vi "Unary ni_measurements_discovery_v1_RegistryService_RegisterService.vi"(8 "error in":errorcluster, 10 "Request Data":T2, 11 "gRPC ID":T5) -> (0 "error out":errorcluster, 2 "Response Data":T1, 3 "gRPC ID out":T5)   [LabVIEW 2020, in "Discovery_client.lvlib"]
uses:
  Discovery_client.lvlib
  <vilib>/gRPC/LabVIEW gRPC Library/Server API/typeDefs/grpcId.ctl
  RPC Messages/ni_measurements_discovery_v1_RegisterServiceRequest.ctl
  RPC Messages/ni_measurements_discovery_v1_ServiceDescriptor.ctl
  RPC Messages/ni_measurements_discovery_v1_ServiceLocation.ctl
  RPC Messages/ni_measurements_discovery_v1_RegisterServiceResponse.ctl
  3477ff3c-ac1a-41b2-98e0-1f89dff8fa77.vi
  <vilib>/gRPC/LabVIEW gRPC Library/Server API/Server/Get Server DLL Path.vi
  <vilib>/gRPC/LabVIEW gRPC Library/Server API/TranslateGrpcError.vi
  <vilib>/gRPC/LabVIEW gRPC Library/gprc-lvsupport-release.lvlib
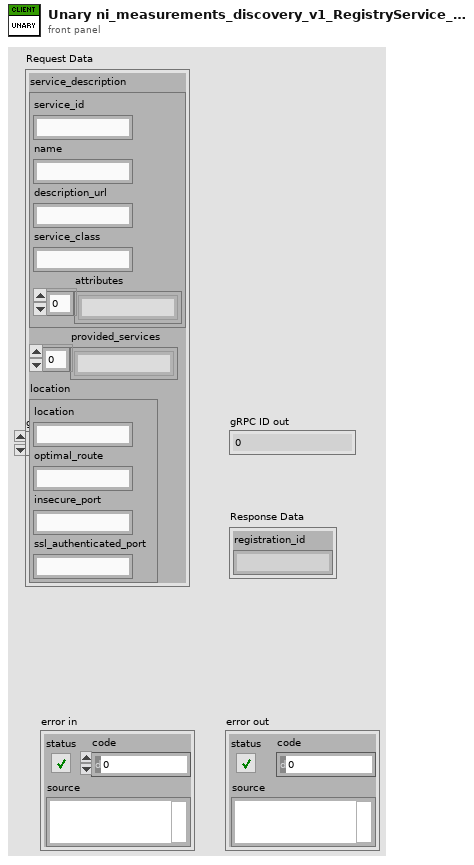
[diagram p1: front panel]
types:
  T1 = typedef "Discovery_client.lvlib/ni_measurements_discovery_v1_RegisterServiceResponse.ctl" = cluster{"registration_id":string}
  T2 = typedef "Discovery_client.lvlib/ni_measurements_discovery_v1_RegisterServiceRequest.ctl" = cluster{"service_description":T3, "provided_services":string[], "location":T4}
  T3 = typedef "Discovery_client.lvlib/ni_measurements_discovery_v1_ServiceDescriptor.ctl" = cluster{"service_id":string, "name":string, "description_url":string, "service_class":string, "attributes":string[]}
  T4 = typedef "Discovery_client.lvlib/ni_measurements_discovery_v1_ServiceLocation.ctl" = cluster{"location":string, "optimal_route":string, "insecure_port":string, "ssl_authenticated_port":string}
  T5 = typedef "gprc-lvsupport-release.lvlib/grpcId.ctl" = u64
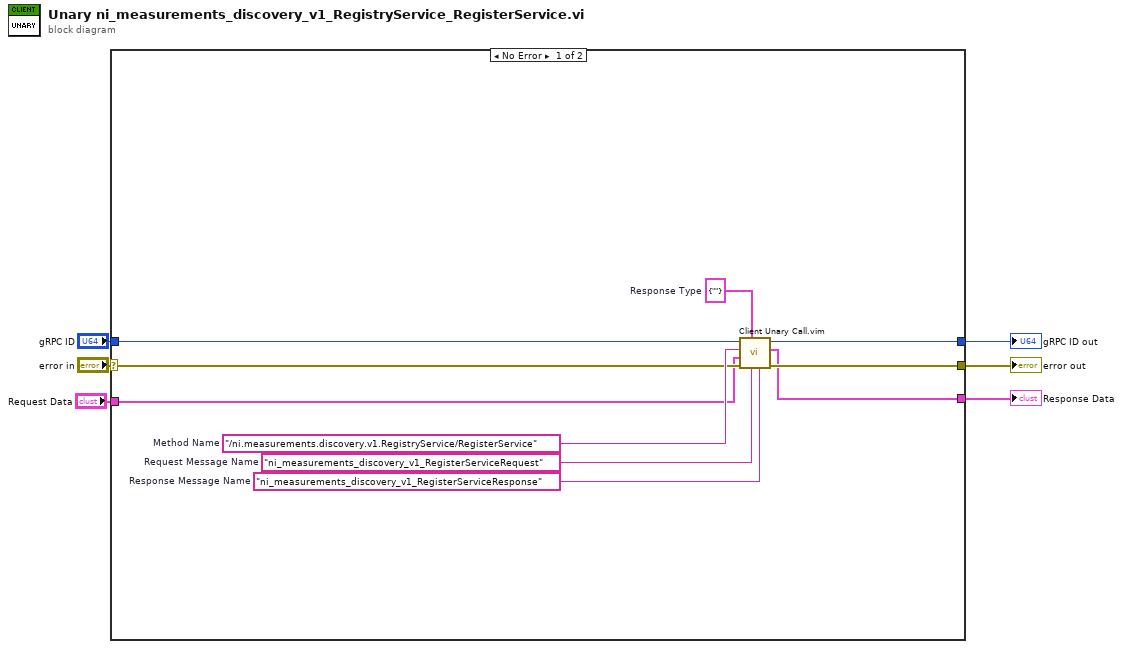
[diagram p0: block diagram]
diagram:
  n1 = case shown="No Error" "error in" {
    selector: "error in" -> [w12 w17]
    tunnel: [w11 w17] -> w5
    tunnel: "gRPC ID" -> [w10 w18]
    tunnel: [w9 w18] -> w3
    tunnel: "Request Data" -> [w8 _]
    tunnel: [w7 _] -> w1
    frame No Error {
      w13 = "ni_measurements_discovery_v1_RegisterServiceResponse"  # Response Message Name
      w14 = "ni_measurements_discovery_v1_RegisterServiceRequest"  # Request Message Name
      w15 = T1 {"registration_id"=""}  # Response Type
      w16 = "/ni.measurements.discovery.v1.RegistryService/RegisterService"  # Method Name
      n2 = call "Client Unary Call.vim"("Response Message Name"=w13, "Request Message Name"=w14, "Response Type"=w15, "error in (no error)"=w12, "Request Data"=w8, "Method Name"=w16, "Client Ref"=w10) -> ("error out"=w11:errorcluster, "Response Data"=w7:T1, "Client Ref Out"=w9:u64)  [unwired: 2 in]
    }
    frame Error {
    }
  }
  "error out" <- w5
  "gRPC ID out" <- w3
  "Response Data" <- w1
